vi "Check Time.vi"(8 "error in (no error)":errorcluster, 11 "DMM Driver in":refnum<class "DMM Driver.lvclass">) -> (0 "error out":errorcluster, 1 "Time OK?":bool, 2 "Remaining Time":i32, 3 "DMM Driver out":refnum<class "DMM Driver.lvclass">)   [LabVIEW 2020, in "DMM.lvlib" / "DMM Driver.lvclass"]
doc: "Evaluate the time elapsed since the start of a measurement. 'Time OK' is set to TRUE if the time has not elapsed."
uses:
  DMM Driver.lvclass
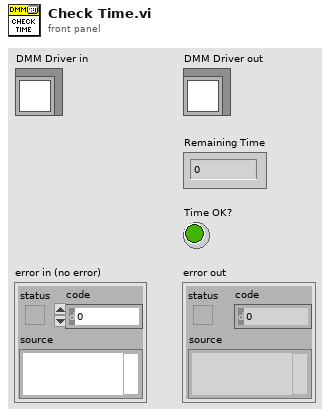
[diagram p1: front panel]
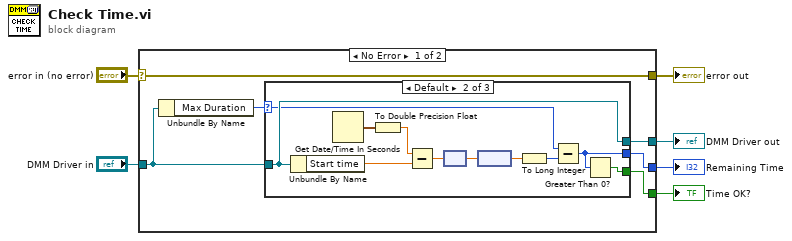
[diagram p0: block diagram]
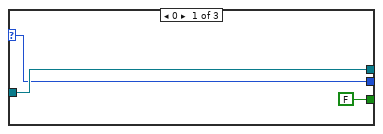
[diagram p2: hidden frame]
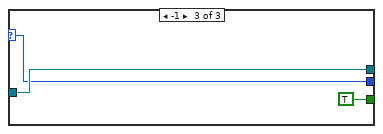
[diagram p3: hidden frame]
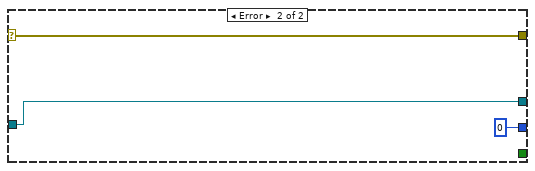
[diagram p4: hidden frame]
diagram:
  n1 = case shown="No Error" "error in (no error)" {
    selector: "error in (no error)" -> [w12 w32]
    tunnel: [w12 w32] -> w5
    tunnel: [w8 w31] -> w3
    tunnel: "DMM Driver in" -> [w9 w31]
    tunnel: [w10 _] -> w2
    tunnel: [w7 0 ("Max Duration")] -> w1
    frame No Error {
      n2 = Unbundle By Name(w9) -> ("Max Duration"=w11:i32)
      n3 = case shown="Default" w11 {
        selector: w11 -> [w13 w20 w27]
        tunnel: [FALSE w18 TRUE] -> w10
        tunnel: [w14 w21 w28] -> w8
        tunnel: w9 -> [w14 w21 w28]
        tunnel: [w13 w17 w27] -> w7
        frame 0 {
        }
        frame Default {
          n4 = Unbundle By Name(w21) -> ("Start time"=w25:dbl)
          n5 = Get Date/Time In Seconds() -> (seconds since 1Jan1904=w26:timestamp)
          n6 = To Double Precision Float(number=w26) -> (double precision float=w16:dbl)
          n7 = Subtract(x=w16, y=w25) -> (x-y=w24:dbl)
          n8 = node(w24) -> (w23:dbl[unit])
          n9 = node(w23) -> (w22:dbl)
          n10 = To Long Integer(number=w22) -> (32bit integer=w19:i32)
          n11 = Subtract(x=w20, y=w19) -> (x-y=w17:i32)
          n12 = Greater Than 0?(x=w17) -> (x > 0?=w18:bool)
        }
        frame -1 {
        }
      }
    }
    frame Error {
    }
  }
  "error out" <- w5
  "DMM Driver out" <- w3
  "Time OK?" <- w2
  "Remaining Time" <- w1
